vi "Configure Control (Numeric).vi"(8 "error in":errorcluster, 10 "control":refnum<vi>, 11 "NT Scalar (Numeric) in":refnum<class "NT Scalar (Numeric).lvclass">) -> (0 "error out":errorcluster, 2 "control out":refnum<vi>, 3 "NT Scalar (Numeric) out":refnum<class "NT Scalar (Numeric).lvclass">)   [LabVIEW 2020, in "PV Access.lvlib" / "PV Data.lvlib" / "NT Scalar (Numeric).lvclass"]
doc: "Set the description, control limits, format and precision of <B>control</B> from the value's metadata."
uses:
  NT Scalar (Numeric).lvclass
  NT Scalar (Numeric).lvclass/NT Scalar (Numeric).ctl
  NT Base/NT Base.lvclass
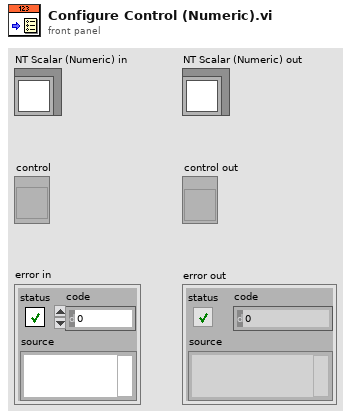
[diagram p1: front panel]
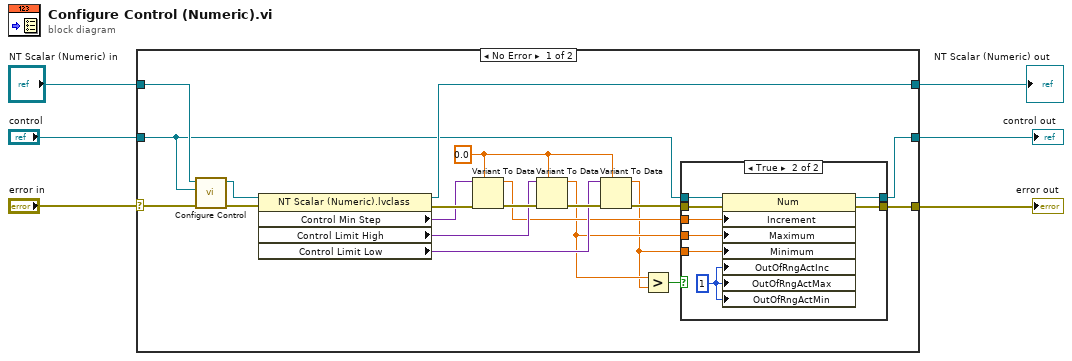
[diagram p0: block diagram]
diagram:
  n1 = case shown="No Error" "error in" {
    selector: "error in" -> [w22 w38]
    tunnel: [w26 w38] -> w6
    tunnel: [w24 w37] -> w5
    tunnel: [w23 w39] -> w4
    tunnel: "NT Scalar (Numeric) in" -> [w21 w39]
    tunnel: "control" -> [w7 w37]
    frame No Error {
      w18 = 0.0
      n2 = call "Configure Control.vi"("error in (no error)"=w22, "control"=w7, "NT Base in"=w21) -> ("error out"=w8:errorcluster, "NT Base out"=w20:refnum<class "NT Scalar (Numeric).lvclass">)  [unwired: 6 in, 1 out]
      n3 = property class="NT Scalar (Numeric).lvclass"(reference=w20, error in=w8) -> (reference out=w23:refnum<class "NT Scalar (Numeric).lvclass">, error out=w19:errorcluster, "Control Min Step"=w15:variant, "Control Limit High"=w14:variant, "Control Limit Low"=w13:variant)
      n4 = Variant To Data(error in=w19, type=w18, Variant=w15) -> (data=w12:dbl, error out=w17:errorcluster)
      n5 = Variant To Data(error in=w17, type=w18, Variant=w14) -> (data=w10:dbl, error out=w16:errorcluster)
      n6 = Variant To Data(error in=w16, type=w18, Variant=w13) -> (data=w9:dbl, error out=w11:errorcluster)
      n7 = Greater?(x=w10, y=w9) -> (0:w25:bool)
      n8 = case shown="True" w25 {
        tunnel: [w28 w36] -> w26
        tunnel: w7 -> [w27 w35]
        tunnel: w12 -> [_ w34]
        tunnel: w10 -> [_ w33]
        tunnel: w9 -> [_ w32]
        tunnel: w11 -> [w28 w31]
        tunnel: [w27 w29] -> w24
        frame False {
        }
        frame True {
          w30 = u8 1 ("Response to Value Outside Limits:Minimum")
          n9 = property on="Property Node" class="Num"(reference=w35, error in=w31, "Increment"=w34, "Maximum"=w33, "Minimum"=w32, "OutOfRngActInc"=w30, "OutOfRngActMax"=w30, "OutOfRngActMin"=w30) -> (reference out=w29:refnum<vi>, error out=w36:errorcluster)
        }
      }
    }
    frame Error {
    }
  }
  "error out" <- w6
  "NT Scalar (Numeric) out" <- w4
  "control out" <- w5
